vi "GetKalmanXY.vi"(1 "KalmanStr":string) -> (0 "kalman_xy":cluster{dbl[], dbl[]})   [LabVIEW 2011]
panel:
  out "x":dbl
  out "y":dbl
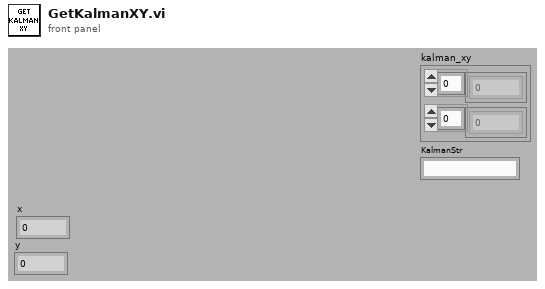
[diagram p1: front panel]
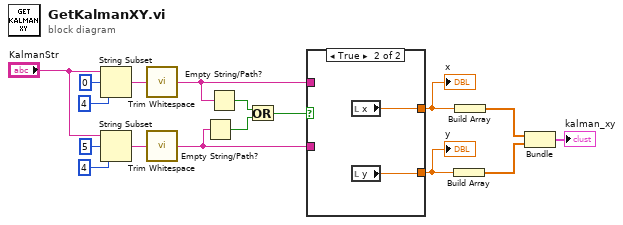
[diagram p0: block diagram]
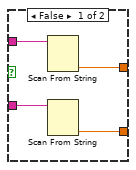
[diagram p2: hidden frame]
diagram:
  n1 = String Subset(string="KalmanStr", offset (0)=0, length (rest)=4 ("length (rest)")) -> (substring=w7:string)
  n2 = String Subset(string="KalmanStr", offset (0)=5, length (rest)=4 ("length (rest)")) -> (substring=w8:string)
  n3 = call <vilib>:"Trim Whitespace.vi"("string"=w7) -> ("trimmed string"=w10:string)  [unwired: 1 in]
  n4 = call <vilib>:"Trim Whitespace.vi"("string"=w8) -> ("trimmed string"=w9:string)  [unwired: 1 in]
  n5 = Empty String/Path?(string/path=w9) -> (empty?=w11:bool)
  n6 = Empty String/Path?(string/path=w10) -> (empty?=w12:bool)
  n7 = Or(x=w12, y=w11) -> (x .or. y?=w13:bool)
  n8 = case shown="True" w13 {
    tunnel: w10 -> [w21 _]
    tunnel: w9 -> [w20 _]
    tunnel: [w19 w23] -> w14
    tunnel: [w18 w22] -> w15
    frame False {
      n9 = Scan From String(input string=w21) -> (output 1=w19:dbl)  [unwired: 4 in, 3 out]
      n10 = Scan From String(input string=w20) -> (output 1=w18:dbl)  [unwired: 4 in, 3 out]
    }
    frame True {
      n11 = local read "x"() -> (w23:dbl)
      n12 = local read "y"() -> (w22:dbl)
    }
  }
  "x" <- w14
  "y" <- w15
  n13 = Build Array(w15) -> (w17:dbl[])
  n14 = Build Array(w14) -> (w16:dbl[])
  n15 = Bundle(w16, w17) -> (→"kalman_xy":cluster{dbl[], dbl[]})  [unwired: 1 in]
